vi "Set Digital Pin Mode b.vi"(0 "Arduino Resource in":T3, 5 "Digital I/O Pin":u8, 9 "Pin Mode (Input)":T4, 11 "error in":errorcluster) -> (4 "Arduino Resource out":T3, 15 "error out":errorcluster)   [LabVIEW 2015]
doc: "Configures the specified digital I/O pin (D0 - D13) as either input or output."
uses:
  <vilib>/LabVIEW Interface for Arduino/Type Defs/Pin Mode.ctl
  <vilib>/LabVIEW Interface for Arduino/Type Defs/Board Type.ctl
  <vilib>/LabVIEW Interface for Arduino/Type Defs/Connection Type.ctl
  <vilib>/LabVIEW Interface for Arduino/Type Defs/Command.ctl
  <vilib>/LabVIEW Interface for Arduino/LabVIEW Interface for Arduino.lvlib
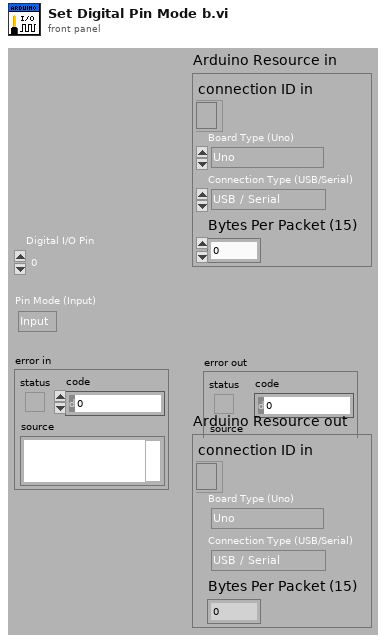
[diagram p1: front panel]
types:
  T1 = typedef "LabVIEW Interface for Arduino.lvlib/Board Type.ctl" = enum16{"Uno", "Dimuelanove w/Atmega 328", "Mega 2560"}
  T2 = typedef "LabVIEW Interface for Arduino.lvlib/Connection Type.ctl" = enum8{"USB / Serial", "XBEE", "BlueSmirf (Bluetooth)"}
  T3 = cluster{"connection ID in":refnum<k31>, "Board Type (Uno)":T1, "Connection Type (USB/Serial)":T2, "Bytes Per Packet (15)":u32}
  T4 = typedef "LabVIEW Interface for Arduino.lvlib/Pin Mode.ctl" = enum8{"Input", "Output"}
  T5 = typedef "LabVIEW Interface for Arduino.lvlib/Command.ctl" = enum8{"setArduinoMode", "flushSerial", "setPinMode", "digitalWritePin", "digitalWritePort", "tone", "digitalReadPin", "digitalReadPort", "analogReadPin", "analogReadPort", "pwmWritePin", "pwmWritePort", "sevenSegment_Configure", "sevenSegment_Write", "I2C Init", "I2C Write", "I2C Read", "SPI Init", "SPI Set Bit Order", "SPI Set Clock Divider", "SPI Set Data Mode", "SPI Send / Receive", "SPI Close", "Servo Set Num Servos", "Servo Config Servo", "Servo Write Angle", "Servo Read Angle", "Servo Write Pulse Width", "Servo Read Pulse Width", "Servo Detach", "LCD Init", "LCD Set Size", "LCD Set Cursor Mode", "LCD Clear", "LCD Set Cursor Position", "LCD Print", "LCD Display Power", "LCD Scroll Display", "LCD Autoscroll", "LCD Print Direction", "LCD Create Custom Char", "LCD Print Custom Char", "contAcqOn", "contAcqOff", "getFirmwareVersion", "FiniteSampleStart"}
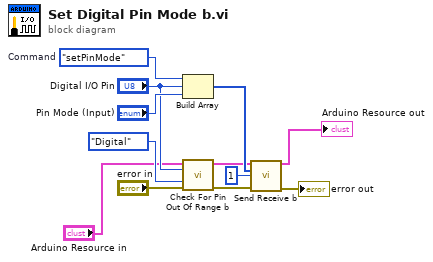
[diagram p0: block diagram]
diagram:
  w12 = Command."setPinMode"  # Command
  n1 = Build Array(w12, "Digital I/O Pin", "Pin Mode (Input)") -> (w7:u8[])
  n2 = call "Check For Pin Out Of Range b.vi"("Arduino Resource in"="Arduino Resource in", "User Pin Number"="Digital I/O Pin", "Pin Type"=enum16{"Analog", "Digital"}."Digital", "error in"="error in") -> ("Arduino Resource out"=w6:T3, "error out"=w5:errorcluster)  [unwired: 10 in]
  n3 = call "Send Receive b.vi"("Arduino Resource"=w6, "Data"=w7, "Bytes To Read (0)"=u8 1, "error in"=w5) -> ("Arduino Resource out"=→"Arduino Resource out":T3, "error out"=→"error out":errorcluster)  [unwired: 9 in, 1 out]
